vi "WSVCAP SHL FPGA LL Procedure RFFE - Send Data.vi"(0 "Procedure Step":T1, 1 "Wait Ticks Remaining":u32, 2 "CMD Length [1-48]":u8, 5 "RFFE Wait Ticks":u32, 7 "Write Bit Index [0-47]":u8, 9 "RFFE Cycle Mode":bool, 11 "error in (no error)":errorcluster, 12 "RFFE Cycle CMD":u64) -> (3 "Wait Ticks Remaining Out":u32, 4 "Procedure Step Out":T1, 8 "Write Bit Index [0-47] Out":u8, 10 "Finished":bool, 15 "error out":errorcluster)   [LabVIEW 2012]
uses:
  Type Defs/WSVCAP SHL Procedure Step Enum.ctl
  Type Defs/WSVCAP SHL RFFE Write Line Enum.ctl
  Type Defs/WSVCAP SHL FIFO Operation Enum.ctl
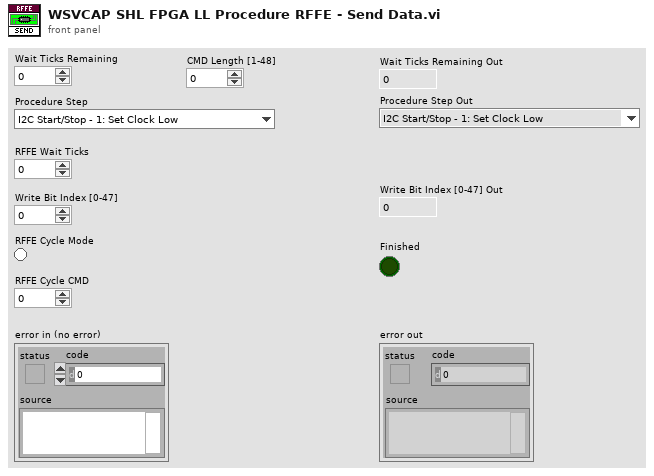
[diagram p1: front panel]
types:
  T1 = typedef "WSVCAP SHL Procedure Step Enum.ctl" = enum16{"I2C Start/Stop - 1: Set Clock Low", "I2C Start/Stop - 2: Wait", "I2C Start/Stop - 3: Set Data I", "I2C Start/Stop - 4: Wait", "I2C Start/Stop - 5: Set Clock High", "I2C Start/Stop - 6: Wait", "I2C Start/Stop - 7: Set Data II", "I2C Start/Stop - 8: Wait", "I2C Start/Stop - 9: Set Clock Low", "I2C Start/Stop - 10: Wait", "I2C Read ACK - 1: Set Clock High", "I2C Read ACK - 2: Wait", "I2C Read ACK - 3: Read ACK Bit", "I2C Read ACK - 4: Wait", "I2C Read ACK - 5: Set Clock Low", "I2C Read ACK - 6: Wait", "I2C Write ACK - 1: Write ACK Bit", "I2C Write ACK - 2: Wait", "I2C Write ACK - 3: Set Clock High", "I2C Write ACK - 4: Wait", "I2C Write ACK - 5: Set Clock Low", "I2C Write ACK - 6: Wait", "I2C Write ACK - 7: Set Data Low", "I2C Send Add - 1: Reset Bits Remaining", "I2C Send Add - 2: Set Data Bit", "I2C Send Add - 3: Wait", "I2C Send Add - 4: Set Clock High", "I2C Send Add - 5: Wait", "I2C Send Add - 6: Set Clock Low", "I2C Send Add - 7: Wait", "I2C Send Add - 8: Check Bits Remaining", "I2C Send Data - 1: Reset Bits Remaining", "I2C Send Data - 2: Load Write Bit from FIFO", "I2C Send Data - 3: Set Data Bit", "I2C Send Data - 4: Wait", "I2C Send Data - 5: Set Clock High", "I2C Send Data - 6: Wait", "I2C Send Data - 7: Set Clock Low", "I2C Send Data - 8: Wait", "I2C Send Data - 9: Check Bits Remaining", "I2C Receive Data - 1: Reset Bits Remaining", "I2C Receive Data - 2: Wait", "I2C Receive Data - 3: Set Clock High", "I2C Receive Data - 4: Wait", "I2C Receive Data - 5: Read Data Bit", "I2C Receive Data - 6: Wait", "I2C Receive Data - 7: Set Clock Low", "I2C Receive Data - 8: Wait", "I2C Receive Data - 9: Check Bits Remaining", "RFFE Send SSC - 1:Set Low", "RFFE Send SSC - 2:Wait", "RFFE Send SSC - 3:Set SDA High", "RFFE Send SSC - 4:Wait", "RFFE Send SSC - 5:Set SDA Low", "RFFE Send SSC - 6:Wait", "RFFE Send Data - 1:Set SCL High", "RFFE Send Data - 2:Wait", "RFFE Send Data - 3:Set SCL Low", "RFFE Send Data - 4:Wait", "RFFE Send Data - 5:Set SCL High (P)", "RFFE Send Data - 6:Wait", "RFFE Send Data - 7:Set SCL Low (P)", "RFFE Send Data - 8:Wait", "RFFE Send Data - 9:Set SCL High (BP)", "RFFE Send Data - 10:Wait", "RFFE Send Data - 11:Set SCL Low (BP)", "RFFE Send Data - 12:Wait", "RFFE Receive Data - 1:Set SCL High", "RFFE Receive Data - 2:Wait", "RFFE Receive Data - 3:Set SCL Low", "RFFE Receive Data - 4:Wait", "RFFE Receive Data - 5:Set SCL High (BP)", "RFFE Receive Data - 6:Wait", "RFFE Receive Data - 7:Set SCL Low (BP)", "RFFE Receive Data - 8:Wait", "RFFE Wait CMD Delay - 1:Wait", "RFFE Clear Lines - 1:Clear"}
  T2 = typedef "WSVCAP SHL RFFE Write Line Enum.ctl" = enum16{"SDAA", "SCLK"}
  T3 = typedef "WSVCAP SHL FIFO Operation Enum.ctl" = enum16{"Create FIFO/Memory", "Get Write FIFO Status", "Get Read FIFO Status", "Put Element in Write", "Put Element in Read", "Get Element from Write", "Get Element from Read"}
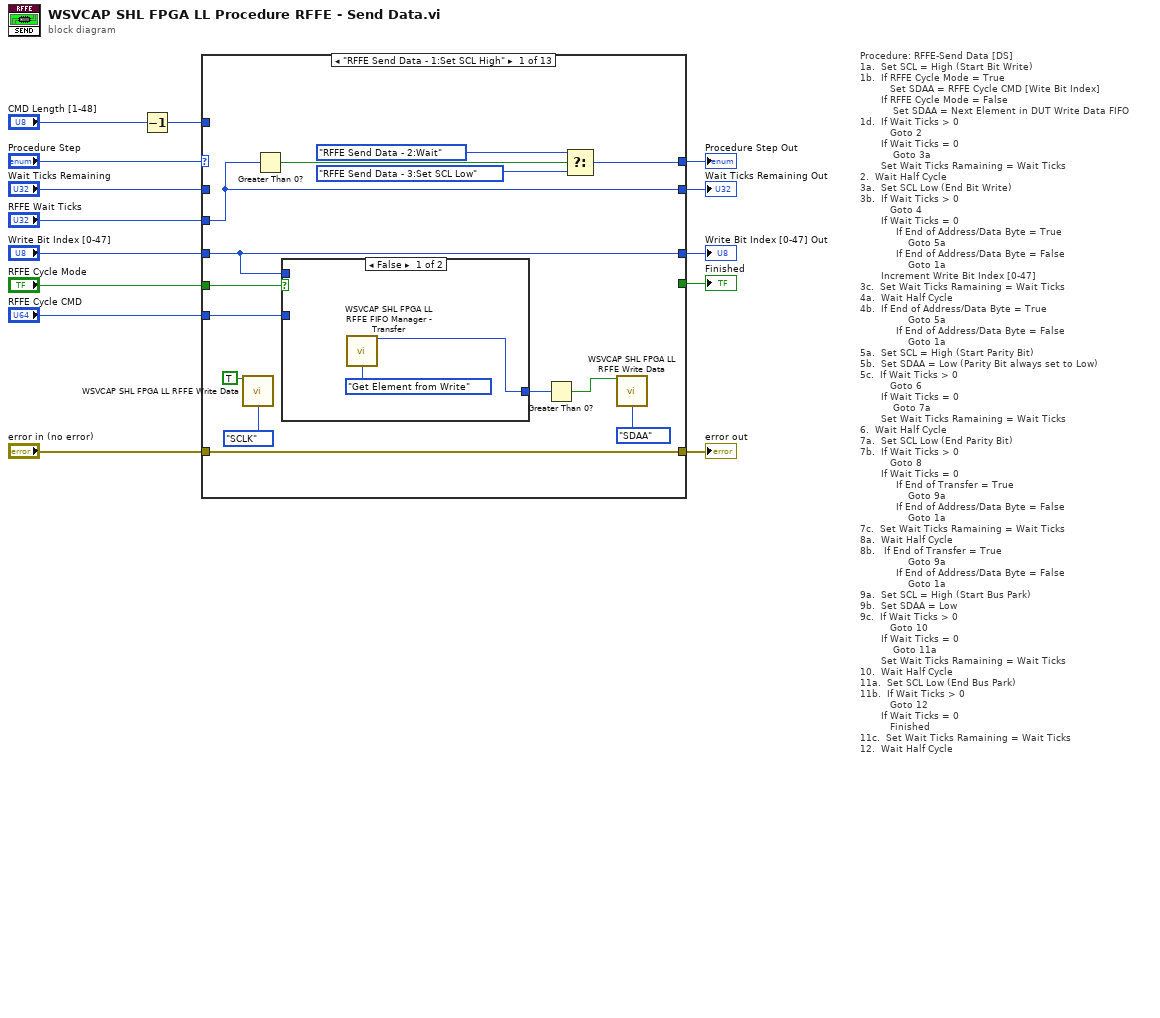
[diagram p0: block diagram]
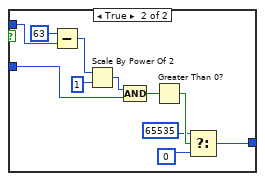
[diagram p2: hidden frame]
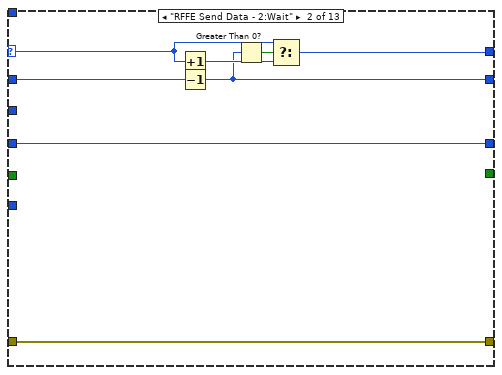
[diagram p3: hidden frame]
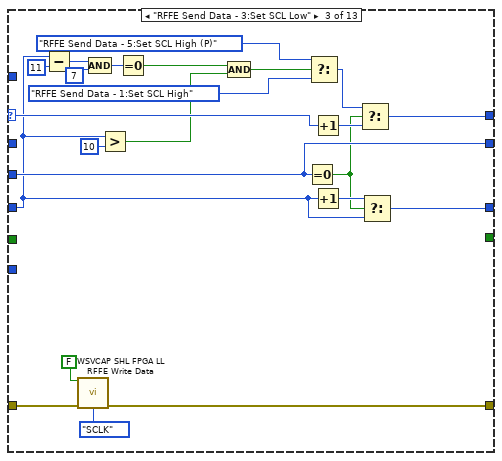
[diagram p4: hidden frame]
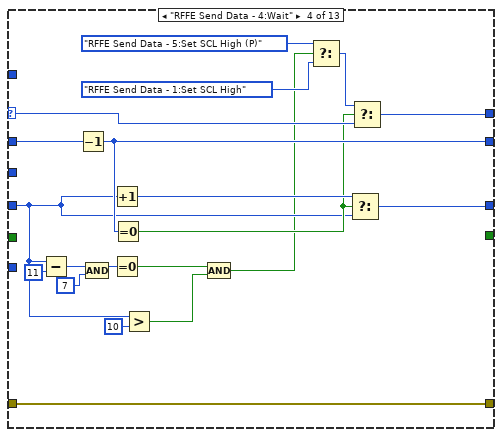
[diagram p5: hidden frame]
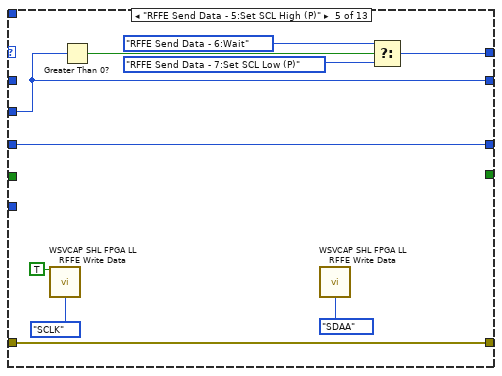
[diagram p6: hidden frame]
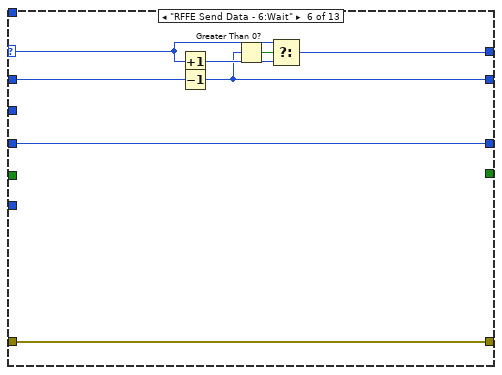
[diagram p7: hidden frame]
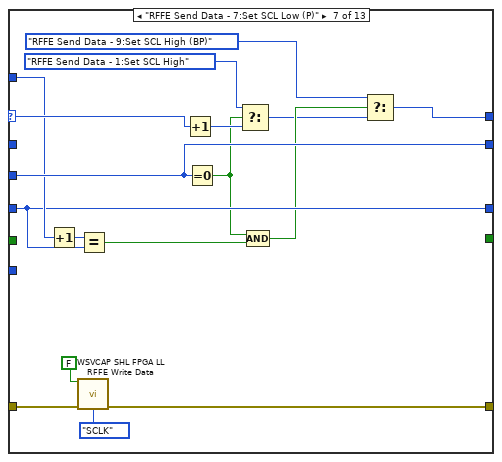
[diagram p8: hidden frame]
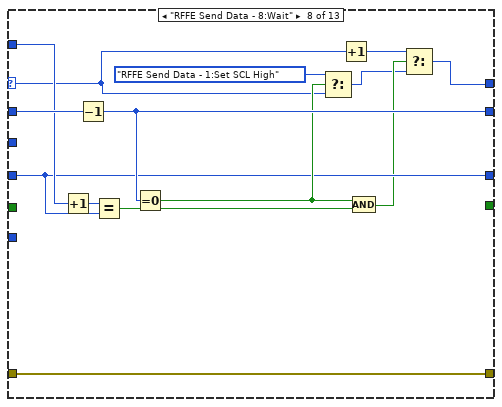
[diagram p9: hidden frame]
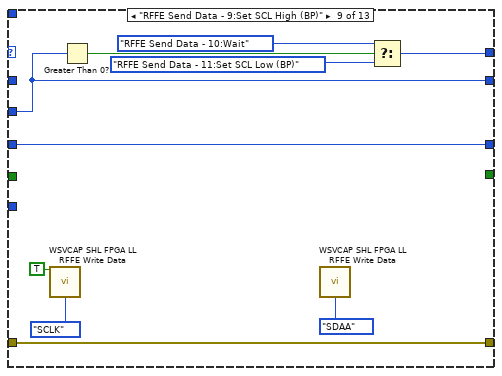
[diagram p10: hidden frame]
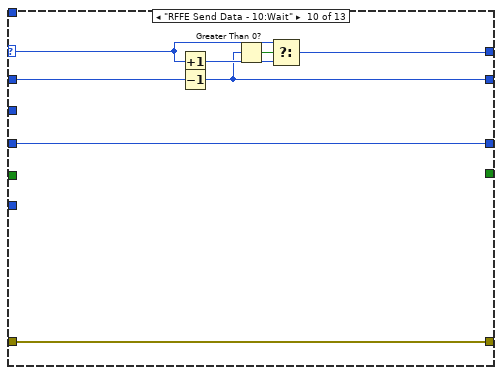
[diagram p11: hidden frame]
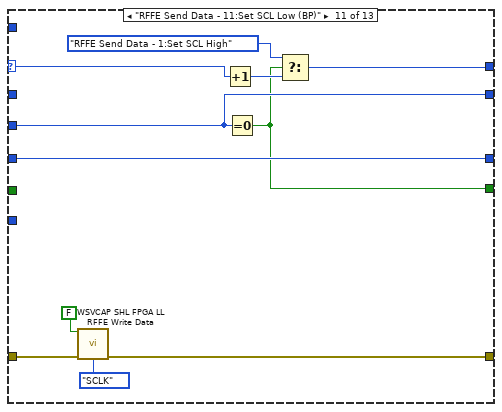
[diagram p12: hidden frame]
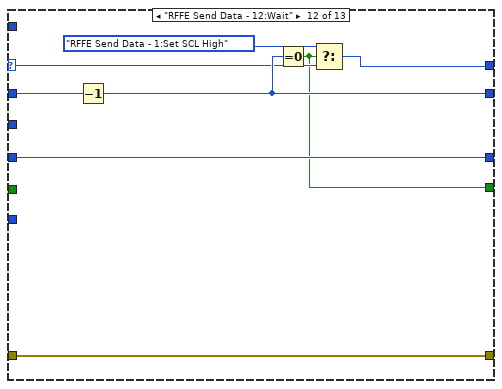
[diagram p13: hidden frame]
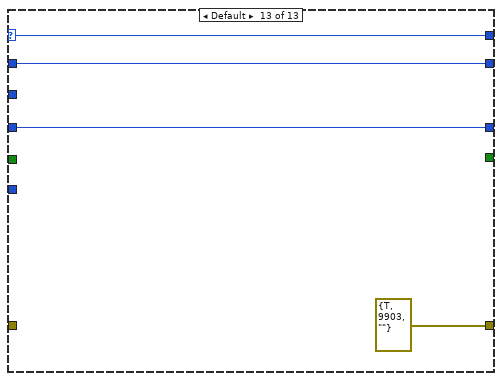
[diagram p14: hidden frame]
diagram:
  # "Procedure: RFFE-Send Data [DS]\n1a.  Set SCL = High (Start Bit Write)\n1b.  If RFFE Cycle Mode = True\n          Set SDAA = RFFE Cycle CMD [Wite Bit Index]\n       If RFFE Cycle Mode = False\n           Set SDAA = Next Element in DUT Write Data FIFO\n1d.  If Wait Ticks > 0\n          Goto 2\n       If Wait Ticks = 0 \n           Goto 3a\n       Set Wait Ticks Ramaining = Wait Ticks\n2.  Wait Half Cycle\n3a.  Set SCL Low (End Bit Write)\n3b.  If Wait Ticks > 0\n          Goto 4\n       If Wait Ticks = 0 \n            If End of Address/Data Byte = True\n                Goto 5a\n            If End of Address/Data Byte = False\n                Goto 1a\n       Increment Write Bit Index [0-47]\n3c.  Set Wait Ticks Ramaining = Wait Ticks     \n4a.  Wait Half Cycle\n4b.  If End of Address/Data Byte = True\n                Goto 5a\n            If End of Address/Data Byte = False\n                Goto 1a\n5a.  Set SCL = High (Start Parity Bit)\n5b.  Set SDAA = Low (Parity Bit always set to Low)\n5c.  If Wait Ticks > 0\n          Goto 6\n       If Wait Ticks = 0 \n           Goto 7a\n       Set Wait Ticks Ramaining = Wait Ticks\n6.  Wait Half Cycle\n7a.  Set SCL Low (End Parity Bit)\n7b.  If Wait Ticks > 0\n          Goto 8\n       If Wait Ticks = 0 \n            If End of Transfer = True\n                Goto 9a\n            If End of Address/Data Byte = False\n                Goto 1a\n7c.  Set Wait Ticks Ramaining = Wait Ticks\n8a.  Wait Half Cycle\n8b.   If End of Transfer = True\n                Goto 9a\n            If End of Address/Data Byte = False\n                Goto 1a\n9a.  Set SCL = High (Start Bus Park)\n9b.  Set SDAA = Low\n9c.  If Wait Ticks > 0\n          Goto 10\n       If Wait Ticks = 0 \n           Goto 11a\n       Set Wait Ticks Ramaining = Wait Ticks\n10.  Wait Half Cycle\n11a.  Set SCL Low (End Bus Park)\n11b.  If Wait Ticks > 0\n          Goto 12\n       If Wait Ticks = 0 \n          Finished\n11c.  Set Wait Ticks Ramaining = Wait Ticks\n12.  Wait Half Cycle"
  n1 = Decrement(x="CMD Length [1-48]") -> (x-1=w1:u8)
  n2 = case shown="\"RFFE Send Data - 1:Set SCL High\"" "Procedure Step" {
    selector: "Procedure Step" -> [_ w47 w72 w91 _ w108 w127 w130 _ w157 w170 w173 w181]
    tunnel: [w24 w49 w67 w92 w98 w110 w122 w141 w147 w159 w165 w178 errorcluster {"status"=TRUE, "code"=9903, "source"=""} ("error IO")] -> w13
    tunnel: "error in (no error)" -> [w24 w49 w68 w92 w98 w110 w123 w141 w147 w159 w166 w178 _]
    tunnel: "Wait Ticks Remaining" -> [_ w45 _ w90 _ w106 _ w140 _ w155 _ w177 w180]
    tunnel: "RFFE Wait Ticks" -> [w18 _ w64 _ w94 _ w121 _ w143 _ w163 _ _]
    tunnel: [_ _ _ _ _ _ _ _ _ _ w160 w171 _] -> w12
    tunnel: "Write Bit Index [0-47]" -> [w17 w42 w57 w79 w93 w103 w118 w135 w142 w152 w161 w174 w179]
    tunnel: "RFFE Cycle Mode" -> [w23 _ _ _ _ _ _ _ _ _ _ _ _]
    tunnel: "RFFE Cycle CMD" -> [w22 _ _ _ _ _ _ _ _ _ _ _ _]
    tunnel: w1 -> [_ _ _ _ _ _ w119 w136 _ _ _ _ _]
    tunnel: [w19 w44 w65 w89 w95 w105 w111 w128 w144 w154 w164 w172 w181] -> w5
    tunnel: [w18 w43 w64 w88 w94 w104 w121 w139 w143 w153 w163 w176 w180] -> w4
    tunnel: [w17 w42 w63 w85 w93 w103 w118 w135 w142 w152 w161 w174 w179] -> w3
    frame "RFFE Send Data - 1:Set SCL High" {
      n3 = call "WSVCAP SHL FPGA LL RFFE Write Data.vi"("Bit In"=TRUE, "Line"=WSVCAP_SHL_RFFE_Write_Line_Enum."SCLK") -> ()  [unwired: 13 in, 1 out]
      n4 = Greater Than 0?(x=w18) -> (x > 0?=w25:bool)
      n5 = case shown="False" w23 {
        tunnel: [w29 w35] -> w16
        tunnel: w22 -> [_ w34]
        tunnel: w17 -> [_ w32]
        frame False {
          n6 = call "WSVCAP SHL FPGA LL RFFE FIFO Manager - Transfer.vi"("Operation"=WSVCAP_SHL_FIFO_Operation_Enum."Get Element from Write") -> ("Data Out"=w29:u64)  [unwired: 12 in, 2 out]
        }
        frame True {
          n7 = Subtract(x=u8 63 ("y"), y=w32) -> (x-y=w31:u8)
          n8 = Scale By Power Of 2(n=w31, x=u64 1 ("Data Out")) -> (x*2^n=w40:u64)
          n9 = Compound Arithmetic op=AND(w40, w34) -> (w39:u64)
          n10 = Greater Than 0?(x=w39) -> (x > 0?=w38:bool)
          n11 = Select(t=u16 65535 ("Data Out"), s=w38, f=u16 0 ("Data Out")) -> (s? t:f=w35:u16)
        }
      }
      n12 = Greater Than 0?(x=w16) -> (x > 0?=w15:bool)
      n13 = Select(t=WSVCAP_SHL_Procedure_Step_Enum."RFFE Send Data - 2:Wait" ("Procedure Step"), s=w25, f=WSVCAP_SHL_Procedure_Step_Enum."RFFE Send Data - 3:Set SCL Low" ("Procedure Step")) -> (s? t:f=w19:T1)
      n14 = call "WSVCAP SHL FPGA LL RFFE Write Data.vi"("Bit In"=w15, "Line"=WSVCAP_SHL_RFFE_Write_Line_Enum."SDAA") -> ()  [unwired: 13 in, 1 out]
    }
    frame "RFFE Send Data - 2:Wait" {
      n15 = Increment(x=w47) -> (x+1=w46:T1)
      n16 = Decrement(x=w45) -> (x-1=w43:u32)
      n17 = Greater Than 0?(x=w43) -> (x > 0?=w48:bool)
      n18 = Select(t=w47, s=w48, f=w46) -> (s? t:f=w44:T1)
    }
    frame "RFFE Send Data - 3:Set SCL Low" {
      n19 = Subtract(x=w57, y=u8 11) -> (x-y=w52:u8)
      n20 = call "WSVCAP SHL FPGA LL RFFE Write Data.vi"("Bit In"=FALSE, "error in (no error)"=w68, "Line"=WSVCAP_SHL_RFFE_Write_Line_Enum."SCLK") -> ("error out"=w67:errorcluster)  [unwired: 12 in]
      n21 = Compound Arithmetic op=AND(w52, u8 7 ("y")) -> (w50:u8)
      n22 = Greater?(x=w57, y=u8 10) -> (0:w54:bool)
      n23 = Equal To 0?(x=w50) -> (x = 0?=w55:bool)
      n24 = Compound Arithmetic op=AND(w55, w54) -> (w53:bool)
      n25 = Equal To 0?(x=w64) -> (x = 0?=w59:bool)
      n26 = Select(t=WSVCAP_SHL_Procedure_Step_Enum."RFFE Send Data - 5:Set SCL High (P)" ("Procedure Step"), s=w53, f=WSVCAP_SHL_Procedure_Step_Enum."RFFE Send Data - 1:Set SCL High" ("Procedure Step")) -> (s? t:f=w60:T1)
      n27 = Increment(x=w72) -> (x+1=w71:T1)
      n28 = Increment(x=w57) -> (x+1=w66:u8)
      n29 = Select(t=w60, s=w59, f=w71) -> (s? t:f=w65:T1)
      n30 = Select(t=w66, s=w59, f=w57) -> (s? t:f=w63:u8)
    }
    frame "RFFE Send Data - 4:Wait" {
      n31 = Subtract(x=w79, y=u8 11) -> (x-y=w75:u8)
      n32 = Decrement(x=w90) -> (x-1=w88:u32)
      n33 = Compound Arithmetic op=AND(w75, u8 7 ("y")) -> (w74:u8)
      n34 = Increment(x=w79) -> (x+1=w87:u8)
      n35 = Equal To 0?(x=w74) -> (x = 0?=w77:bool)
      n36 = Equal To 0?(x=w88) -> (x = 0?=w86:bool)
      n37 = Greater?(x=w79, y=u8 10) -> (0:w78:bool)
      n38 = Compound Arithmetic op=AND(w77, w78) -> (w76:bool)
      n39 = Select(t=WSVCAP_SHL_Procedure_Step_Enum."RFFE Send Data - 5:Set SCL High (P)" ("Procedure Step"), s=w76, f=WSVCAP_SHL_Procedure_Step_Enum."RFFE Send Data - 1:Set SCL High" ("Procedure Step")) -> (s? t:f=w82:T1)
      n40 = Select(t=w87, s=w86, f=w79) -> (s? t:f=w85:u8)
      n41 = Select(t=w82, s=w86, f=w91) -> (s? t:f=w89:T1)
    }
    frame "RFFE Send Data - 5:Set SCL High (P)" {
      n42 = call "WSVCAP SHL FPGA LL RFFE Write Data.vi"("Bit In"=TRUE, "Line"=WSVCAP_SHL_RFFE_Write_Line_Enum."SCLK") -> ()  [unwired: 13 in, 1 out]
      n43 = Greater Than 0?(x=w94) -> (x > 0?=w99:bool)
      n44 = call "WSVCAP SHL FPGA LL RFFE Write Data.vi"("Line"=WSVCAP_SHL_RFFE_Write_Line_Enum."SDAA") -> ()  [unwired: 14 in, 1 out]
      n45 = Select(t=WSVCAP_SHL_Procedure_Step_Enum."RFFE Send Data - 6:Wait" ("Procedure Step"), s=w99, f=WSVCAP_SHL_Procedure_Step_Enum."RFFE Send Data - 7:Set SCL Low (P)" ("Procedure Step")) -> (s? t:f=w95:T1)
    }
    frame "RFFE Send Data - 6:Wait" {
      n46 = Increment(x=w108) -> (x+1=w107:T1)
      n47 = Decrement(x=w106) -> (x-1=w104:u32)
      n48 = Greater Than 0?(x=w104) -> (x > 0?=w109:bool)
      n49 = Select(t=w108, s=w109, f=w107) -> (s? t:f=w105:T1)
    }
    frame "RFFE Send Data - 7:Set SCL Low (P)" {
      n50 = Increment(x=w119) -> (x+1=w115:u8)
      n51 = call "WSVCAP SHL FPGA LL RFFE Write Data.vi"("Bit In"=FALSE, "error in (no error)"=w123, "Line"=WSVCAP_SHL_RFFE_Write_Line_Enum."SCLK") -> ("error out"=w122:errorcluster)  [unwired: 12 in]
      n52 = Equal?(x=w115, y=w118) -> (x = y?=w116:bool)
      n53 = Increment(x=w127) -> (x+1=w126:T1)
      n54 = Equal To 0?(x=w121) -> (x = 0?=w117:bool)
      n55 = Select(t=WSVCAP_SHL_Procedure_Step_Enum."RFFE Send Data - 1:Set SCL High" ("Procedure Step"), s=w117, f=w126) -> (s? t:f=w113:T1)
      n56 = Compound Arithmetic op=AND(w117, w116) -> (w114:bool)
      n57 = Select(t=WSVCAP_SHL_Procedure_Step_Enum."RFFE Send Data - 9:Set SCL High (BP)" ("Procedure Step"), s=w114, f=w113) -> (s? t:f=w111:T1)
    }
    frame "RFFE Send Data - 8:Wait" {
      n58 = Increment(x=w136) -> (x+1=w133:u8)
      n59 = Decrement(x=w140) -> (x-1=w139:u32)
      n60 = Equal?(x=w133, y=w135) -> (x = y?=w134:bool)
      n61 = Equal To 0?(x=w139) -> (x = 0?=w137:bool)
      n62 = Select(t=WSVCAP_SHL_Procedure_Step_Enum."RFFE Send Data - 1:Set SCL High" ("Procedure Step"), s=w137, f=w130) -> (s? t:f=w131:T1)
      n63 = Increment(x=w130) -> (x+1=w129:T1)
      n64 = Compound Arithmetic op=AND(w137, w134) -> (w132:bool)
      n65 = Select(t=w129, s=w132, f=w131) -> (s? t:f=w128:T1)
    }
    frame "RFFE Send Data - 9:Set SCL High (BP)" {
      n66 = call "WSVCAP SHL FPGA LL RFFE Write Data.vi"("Bit In"=TRUE, "Line"=WSVCAP_SHL_RFFE_Write_Line_Enum."SCLK") -> ()  [unwired: 13 in, 1 out]
      n67 = Greater Than 0?(x=w143) -> (x > 0?=w148:bool)
      n68 = call "WSVCAP SHL FPGA LL RFFE Write Data.vi"("Line"=WSVCAP_SHL_RFFE_Write_Line_Enum."SDAA") -> ()  [unwired: 14 in, 1 out]
      n69 = Select(t=WSVCAP_SHL_Procedure_Step_Enum."RFFE Send Data - 10:Wait" ("Procedure Step"), s=w148, f=WSVCAP_SHL_Procedure_Step_Enum."RFFE Send Data - 11:Set SCL Low (BP)" ("Procedure Step")) -> (s? t:f=w144:T1)
    }
    frame "RFFE Send Data - 10:Wait" {
      n70 = Increment(x=w157) -> (x+1=w156:T1)
      n71 = Decrement(x=w155) -> (x-1=w153:u32)
      n72 = Greater Than 0?(x=w153) -> (x > 0?=w158:bool)
      n73 = Select(t=w157, s=w158, f=w156) -> (s? t:f=w154:T1)
    }
    frame "RFFE Send Data - 11:Set SCL Low (BP)" {
      n74 = call "WSVCAP SHL FPGA LL RFFE Write Data.vi"("Bit In"=FALSE, "error in (no error)"=w166, "Line"=WSVCAP_SHL_RFFE_Write_Line_Enum."SCLK") -> ("error out"=w165:errorcluster)  [unwired: 12 in]
      n75 = Increment(x=w170) -> (x+1=w169:T1)
      n76 = Equal To 0?(x=w163) -> (x = 0?=w160:bool)
      n77 = Select(t=WSVCAP_SHL_Procedure_Step_Enum."RFFE Send Data - 1:Set SCL High" ("Procedure Step"), s=w160, f=w169) -> (s? t:f=w164:T1)
    }
    frame "RFFE Send Data - 12:Wait" {
      n78 = Decrement(x=w177) -> (x-1=w176:u32)
      n79 = Equal To 0?(x=w176) -> (x = 0?=w171:bool)
      n80 = Select(t=WSVCAP_SHL_Procedure_Step_Enum."RFFE Send Data - 1:Set SCL High" ("Procedure Step"), s=w171, f=w173) -> (s? t:f=w172:T1)
    }
    frame Default {
    }
  }
  "error out" <- w13
  "Finished" <- w12
  "Procedure Step Out" <- w5
  "Wait Ticks Remaining Out" <- w4
  "Write Bit Index [0-47] Out" <- w3
